vi "GOMDBTS2048 read Calibration Entry Info.vi"(8 "error in (no error)":errorcluster, 10 "calibrationEntryNumber":i32, 11 "handle":i32) -> (0 "error out":errorcluster, 2 "function return":i32, 3 "calibrationName":string)   [LabVIEW 2015, in "GOMDBTS2048.lvlib"]
doc: "GOBTS2048DLL int __stdcall GOMDBTS2048_readCalibrationEntryInfo(int handle, int calibrationEntryNumber, char* calibrationName);"
uses:
  GOMDBTS2048.lvlib
  runtime/GOMDBTS2048.dll
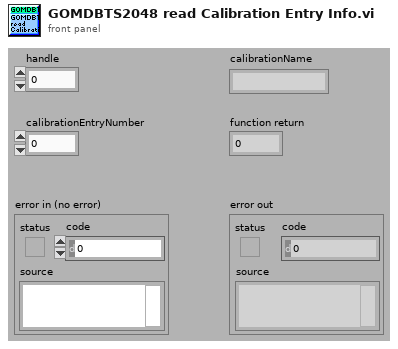
[diagram p1: front panel]
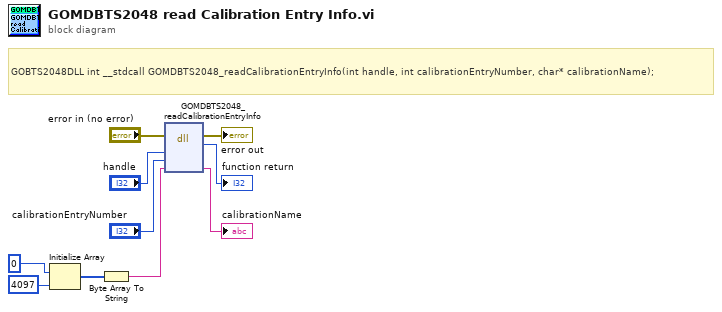
[diagram p0: block diagram]
diagram:
  # "GOBTS2048DLL int __stdcall GOMDBTS2048_readCalibrationEntryInfo(int handle, int calibrationEntryNumber, char* calibrationName);"
  n1 = Initialize Array(u8 0 ("element"), 4097 ("dimension size")) -> (w7:u8[])
  n2 = Byte Array To String(unsigned byte array=w7) -> (string=w6:string)
  n3 = dll-call lib="C:/Users/rkoch/Documents/GO_Library/runtime/GOMDBTS2048.*" fn="GOMDBTS2048_readCalibrationEntryInfo"(error in="error in (no error)", "handle"="handle", "calibrationEntryNumber"="calibrationEntryNumber", "calibrationName"=w6) -> (error out=→"error out":errorcluster, →"function return":i32, "calibrationName"=→"calibrationName":string)  [unwired: 4 in, 1 out]
